vi "format set font shadow.vi"(8 "error in (no error)":errorcluster, 11 "format":u32) -> (0 "error out":errorcluster)   [LabVIEW 2015, in "xlsxwriter.lvlib"]
doc: "void format_set_font_shadow(lxw_format format);"
uses:
  xlsxwriter.lvlib
  xlsxwriter.dll
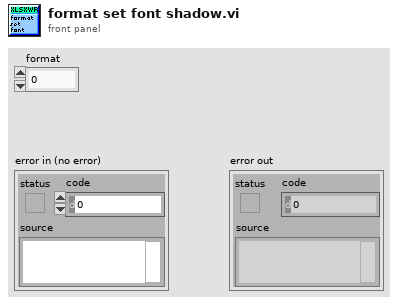
[diagram p1: front panel]
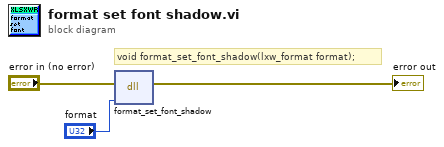
[diagram p0: block diagram]
diagram:
  # "void format_set_font_shadow(lxw_format format);"
  n1 = dll-call lib="C:/Users/WDAGUtilityAccount/Desktop/lv_vis_added_cell/xlsxwriter.*" fn="format_set_font_shadow"(error in="error in (no error)", "format"="format") -> (error out=→"error out":errorcluster)  [unwired: 4 in, 1 out]
